vi "RSZVB Set Power Loss List Trace.vi"(8 "error in (no error)":errorcluster {"code" format="%.0x"}, 9 "Trace Name (\"\")":string, 11 "VISA session":refnum<visa-resource-name>) -> (0 "error out":errorcluster {"code" format="%.0x"}, 3 "dup VISA session":refnum<visa-resource-name>)   [LabVIEW 2011]
doc: "This VI Selects a trace which provides the points for the power loss list.\n\nRemote-control command(s):\nSOURce<Ch>:POWer<Pt>:CORRection:TCOefficient:FEED '<trace_name>'"
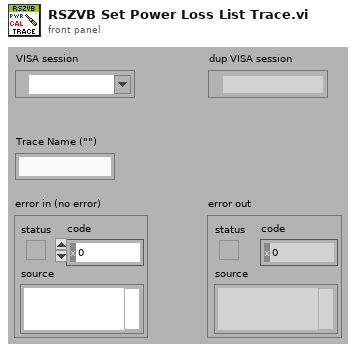
[diagram p1: front panel]
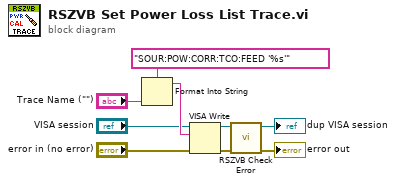
[diagram p0: block diagram]
diagram:
  n1 = Format Into String(format string="SOUR:POW:CORR:TCO:FEED '%s'", "Trace Name (\"\")") -> (resulting string=w6:string)  [unwired: 2 in, 1 out]
  n2 = VISA Write(VISA resource name="VISA session", write buffer=w6, error in (no error)="error in (no error)") -> (VISA resource name out=w7:refnum<visa-resource-name>, error out=w8:errorcluster)  [unwired: 1 out]
  n3 = call "RSZVB Check Error.vi"("error in (no error)"=w8, "VISA session"=w7) -> ("error out"=→"error out":errorcluster, "dup VISA session"=→"dup VISA session":refnum<visa-resource-name>)  [unwired: 8 in]
